vi "Model1.vi"(9 "Switch":bool, 10 "Channel B":dbl, 11 "Channel A":dbl) -> (3 "Output Signal":dbl)   [LabVIEW 2019]
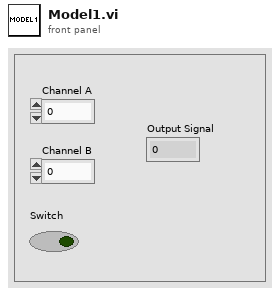
[diagram p1: front panel]
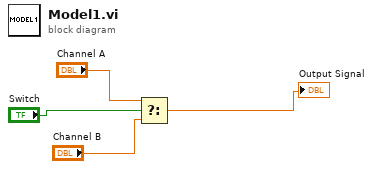
[diagram p0: block diagram]
diagram:
  n1 = Select(t="Channel A", s="Switch", f="Channel B") -> (s? t:f=→"Output Signal":dbl)
